vi "getCategoryUpdateQuery.vi"(8 "error in (no error)":errorcluster, 10 "Category ID":string, 11 "Banking Transaction in":refnum<class "Banking Transaction.lvclass">) -> (0 "error out":errorcluster, 2 "Update Query":string, 3 "Banking Transaction out":refnum<class "Banking Transaction.lvclass">)   [LabVIEW 2018, in "Banking Transaction.lvclass"]
uses:
  Banking Transaction.lvclass
  Transaction/Transaction.lvclass
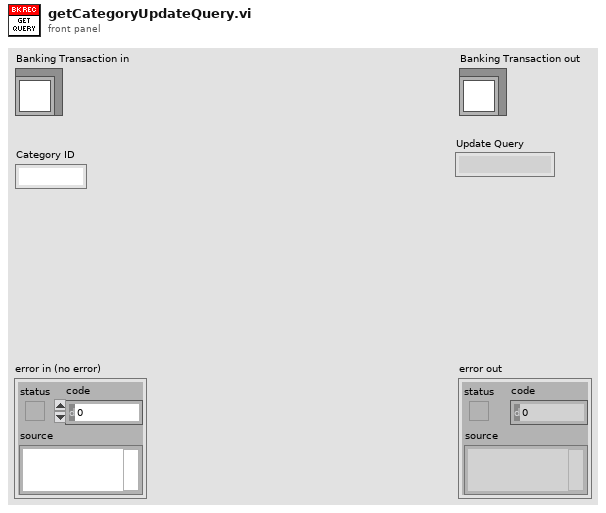
[diagram p1: front panel]
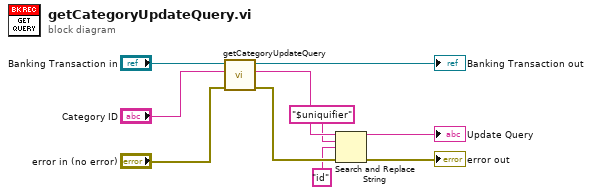
[diagram p0: block diagram]
diagram:
  n1 = call-parent "getCategoryUpdateQuery.vi"("error in (no error)"="error in (no error)", "Category ID"="Category ID", "Transaction in"="Banking Transaction in") -> ("error out"=w6:errorcluster, "Update Query"=w4:string, "Transaction out"=→"Banking Transaction out":refnum<class "Banking Transaction.lvclass">)  [unwired: 6 in]
  n2 = Search and Replace String(input string=w4, search string="$uniquifier", replace string="id" ("replace string (\"\")"), error in=w6) -> (result string=→"Update Query":string, error out=→"error out":errorcluster)  [unwired: 4 in, 2 out]
